vi "Write Characters To File with Advisory Dialog Option with Pattern.vi"(0 "advisory dialog? (display:T)":bool=TRUE, 1 "pattern":string, 6 "append to file? (new file:F)":bool, 9 "character string":string, 11 "file path (dialog if empty)":path) -> (3 "new file path (Not A Path if cancelled)":path, 4 "File Open?":bool=TRUE)   [LabVIEW 2023]
doc: "Writes a character string to a new byte stream file or appends the string to an existing file. The VI opens or creates the file beforehand and closes it afterwards.\n\nfile path is the path name of the file. If file path is empty (default value) or is Not A Path, the VI displays a File dialog box from which you can select a file. Error 43 occurs if the user cancels the dialog. \n\ncharacter string is the data the VI writes to the file.\n\nappend to file? Set to TRUE if you want to append the data to a existing file; you can also set it TRUE to write to a new file. Set to FALSE (default value) if you want to write the data to a new file or to replace an existing file.\n\nnew file path is the path of the file to which the VI wrote data. You can use this output to determine the path of a file that you open using dialog. new file path returns Not A Path if the user selects Cancel from the dialog box."
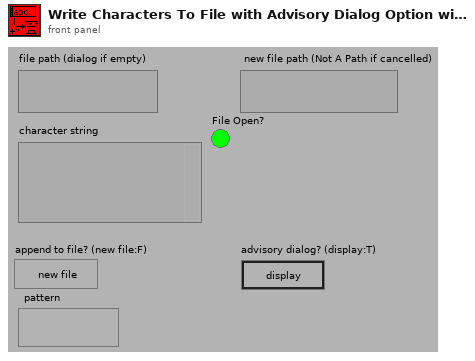
[diagram p1: front panel]
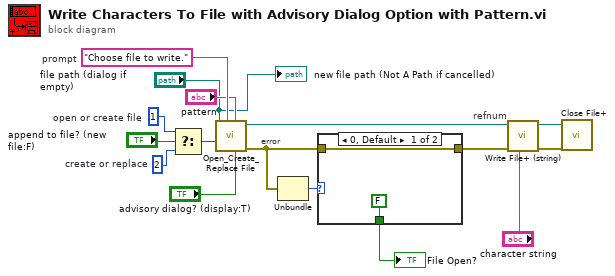
[diagram p0: block diagram]
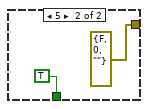
[diagram p2: hidden frame]
diagram:
  w9 = i16 2  # create or replace
  w14 = "Choose file to write."  # prompt
  w12 = i16 1  # open or create file
  # "error"
  # "refnum"
  n1 = Select(t=w12, s="append to file? (new file:F)", f=w9) -> (s? t:f=w13:i16)
  n2 = call <vilib>:"Open_Create_Replace File.vi"("advisory dialog? (display:T)"="advisory dialog? (display:T)", "pattern"="pattern", "prompt"=w14, "function (open:0)"=w13, "file path"="file path (dialog if empty)") -> ("error out"=w4:errorcluster, "refnum"=w8:refnum<file>)  [unwired: 3 in, 2 out]
  n3 = Unbundle(w4) -> ("code"=w5:i32)  [unwired: 2 out]
  n4 = case shown="0, Default" w5 {
    tunnel: w4 -> [w18 _]
    tunnel: [w18 errorcluster {"status"=FALSE, "code"=0, "source"=""} ("error in (no error)")] -> w3
    tunnel: [FALSE TRUE] -> w1
    frame 0, Default {
    }
    frame 5 {
    }
  }
  "File Open?" <- w1
  n5 = call <vilib>:"Write File+ (string).vi"("string"="character string", "error in (no error)"=w3, "refnum"=w8) -> ("error out"=w16:errorcluster, "dup refnum"=w15:refnum<file>)  [unwired: 4 in, 1 out]
  n6 = call <vilib>:"Close File+.vi"("error in (no error)"=w16, "refnum"=w15) -> ()  [unwired: 3 in, 3 out]
  "new file path (Not A Path if cancelled)" <- "file path (dialog if empty)"
